vi "Send.vi"(5 "SentData":string, 6 "Timeout ms":i32, 7 "UDP Input":T1) -> (0 "Error Out":errorcluster, 3 "UDP Output":T1)   [LabVIEW 2019]
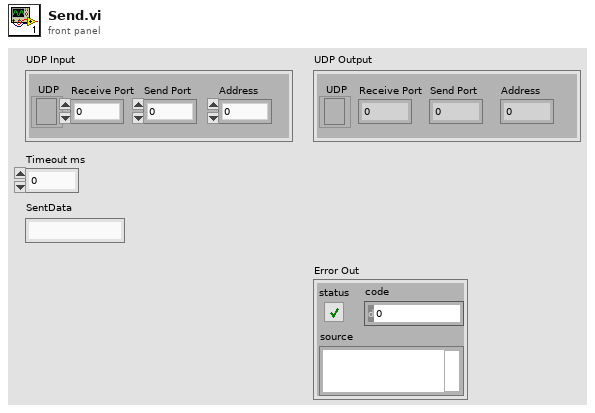
[diagram p1: front panel]
types:
  T1 = cluster{"UDP":refnum<k16>, "Receive Port":i32, "Send Port":i32, "Address":i64}
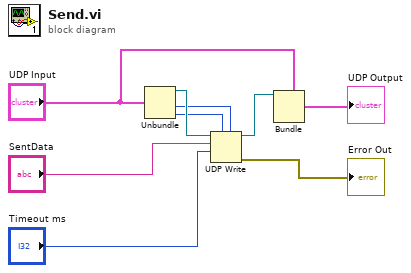
[diagram p0: block diagram]
diagram:
  n1 = Unbundle("UDP Input") -> ("UDP"=w9:refnum<k16>, "Send Port"=w2:i32, "Address"=w8:i64)  [unwired: 1 out]
  n2 = UDP Write(address=w8, port or service name=w2, connection ID=w9, data in="SentData", 9:"Timeout ms") -> (error out=→"Error Out":errorcluster, 3:w5:refnum<k16>)  [unwired: 1 in]
  n3 = Bundle(cluster="UDP Input", "UDP"=w5) -> (→"UDP Output":T1)  [unwired: 3 in]
